vi "DiffDriveTrainSim_CreateKitbotSim_EstMass.vi"(5 "j_KgM2":dbl=1.0, 6 "MeasurementStdDev":T4, 8 "TrackWidth_M":dbl, 9 "Wheelsize":T1, 10 "ToughBoxMiniGear":T2, 11 "ToughBoxMiniMotor":T3) -> (0 "Size Coerced":bool, 3 "DiffDriveTrainSim":T5 {"m_Motor"."Jr_KgM2" format="%13.5p"; "m_Motor"."L_H" format="%13.5p"; "m_Motor"."Kt_NMPerAmp" format="%13.5p"; "m_Motor"."KvINV_RadPerSecPerVolt" format="%13.5p"; "m_Motor"."R_Ohms" format="%13.5p"; "m_Motor"."FreeSpeed_RadPerSec" format="%13.5p"; "m_Motor"."FreeCurrent_Amps" format="%13.5p"; "m_Motor"."StallCurrent_Amps" format="%13.5p"; "m_Motor"."StallTorque_NM" format="%13.5p"; "m_Motor"."nominalVoltage_Volts" format="%13.5p"})   [LabVIEW 2019, in "Trajectory_Library.lvlib"]
doc: "Create a sim for the standard FRC kitbot.\n\nThe mass of the robot is estimated at 25 pounds, converted to kg before use.\n \nInputs:\n - jKgMetersSquared -- The moment of inertia of the drivebase. This can be calculated using SysId.\n - motor -- The motors installed in the bot.\n - gearing -- The gearing reduction used.\n - wheelSize -- The wheel size.\n - trackWidth -- Width between left and right wheels - Meters\n - measurementStdDevs -- Standard deviations for measurements, in the form [x, y, heading, left velocity, right velocity, left distance, right distance]?. Can be null if no noise is desired. Gyro standard deviations of 0.0001 radians, velocity standard deviations of 0.05 m/s, and position measurement standard deviations of 0.005 meters are a reasonable starting point.\n\nOutputs:\n - OutDiffDriveTraimSim -- Updated data cluster.\n - SizeCoerced -- If TRUE, an error occured. Execution may continue"
uses:
  Trajectory_Library.lvlib
  TypeDef/DIFF_DRIVE_TRAIN_SIM.ctl
  TypeDef/LINEAR_SYSTEM.ctl
  <vilib>/Analysis/Matrix/Datatypes/RealMatrix.ctl
  TypeDef/DCMOTOR.CTL
  Enum/DIFF_DRIVE_ToughBoxMini_MotorChoice_ENUM.ctl
  Enum/DIFF_DRIVE_ToughBoxMini_GearChoice_ENUM.ctl
  Enum/DIFF_DRIVE_KitBot_WheelSize_ENUM.ctl
  <vilib>/Analysis/Matrix/NI_Matrix.lvlib
panel:
  # "<1, 1>"
  # "<States, 1>"
  # "<Outputs, 1>"
  # "<Inputs, 1>"
  # "<Outputs, 1>"
  # "<States,States>"
  # "<States,Inputs>"
  # "<Outputs,States>"
  # "<Outputs,Inputs>"
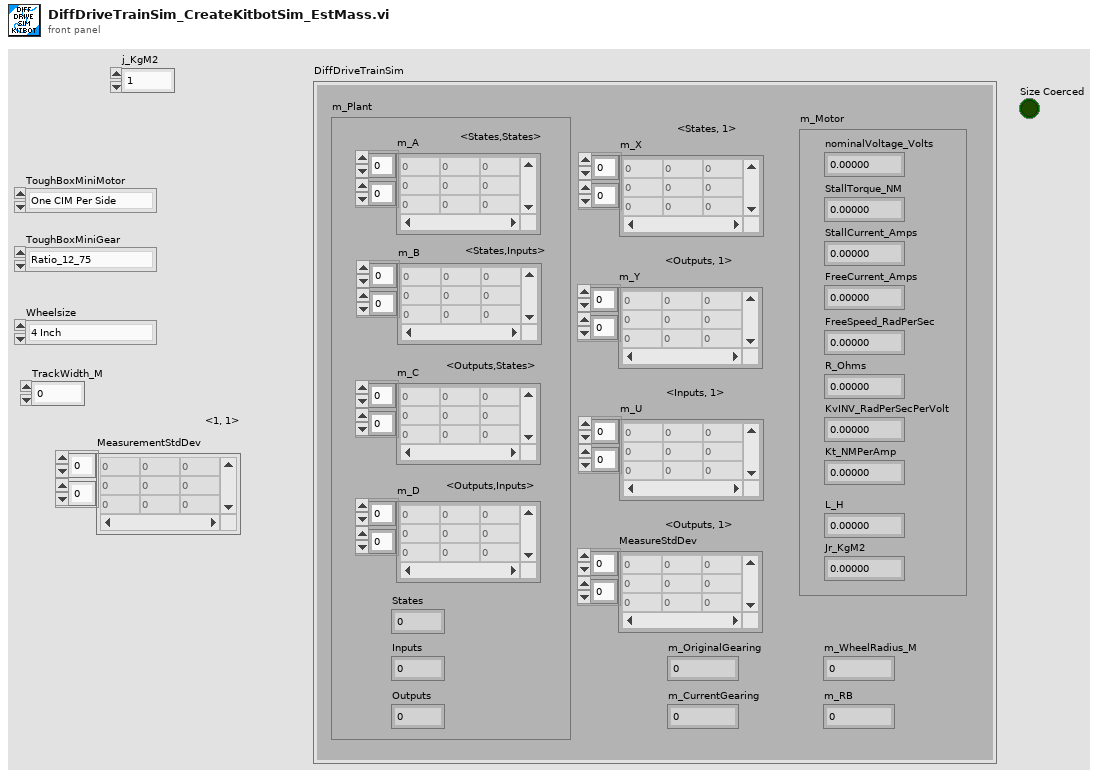
[diagram p1: front panel]
types:
  T1 = typedef "Trajectory_Library.lvlib/DIFF_DRIVE_KitBot_WheelSize_ENUM.ctl" = enum16{"4 Inch", "6 Inch", "8 Inch", "10 Inch"}
  T2 = typedef "Trajectory_Library.lvlib/DIFF_DRIVE_ToughBoxMini_GearChoice_ENUM.ctl" = enum16{"Ratio_12_75", "Ratio_10_71", "Ratio_8_45", "Ratio_7_31", "Ratio_5_95"}
  T3 = typedef "Trajectory_Library.lvlib/DIFF_DRIVE_ToughBoxMini_MotorChoice_ENUM.ctl" = enum16{"One CIM Per Side", "Two CIM Per Side", "One MiniCIM Per Side", "Two Mini CIM Per Side", "Two Falcon Per Side", "Two NEO Per Side"}
  T4 = typedef "NI_Matrix.lvlib/RealMatrix.ctl" = dbl[][]
  T5 = typedef "Trajectory_Library.lvlib/DIFF_DRIVE_TRAIN_SIM.ctl" = cluster{"m_Plant":T6, "m_X":T4, "m_Y":T4, "m_U":T4, "MeasureStdDev":T4, "m_Motor":T7, "m_OriginalGearing":dbl, "m_CurrentGearing":dbl, "m_WheelRadius_M":dbl, "m_RB":dbl}
  T6 = typedef "Trajectory_Library.lvlib/LINEAR_SYSTEM.ctl" = cluster{"m_A":T4, "m_B":T4, "m_C":T4, "m_D":T4, "States":i32, "Inputs":i32, "Outputs":i32}
  T7 = typedef "Trajectory_Library.lvlib/DCMOTOR.CTL" = cluster{"nominalVoltage_Volts":dbl, "StallTorque_NM":dbl, "StallCurrent_Amps":dbl, "FreeCurrent_Amps":dbl, "FreeSpeed_RadPerSec":dbl, "R_Ohms":dbl, "KvINV_RadPerSecPerVolt":dbl, "Kt_NMPerAmp":dbl, "L_H":dbl, "Jr_KgM2":dbl}
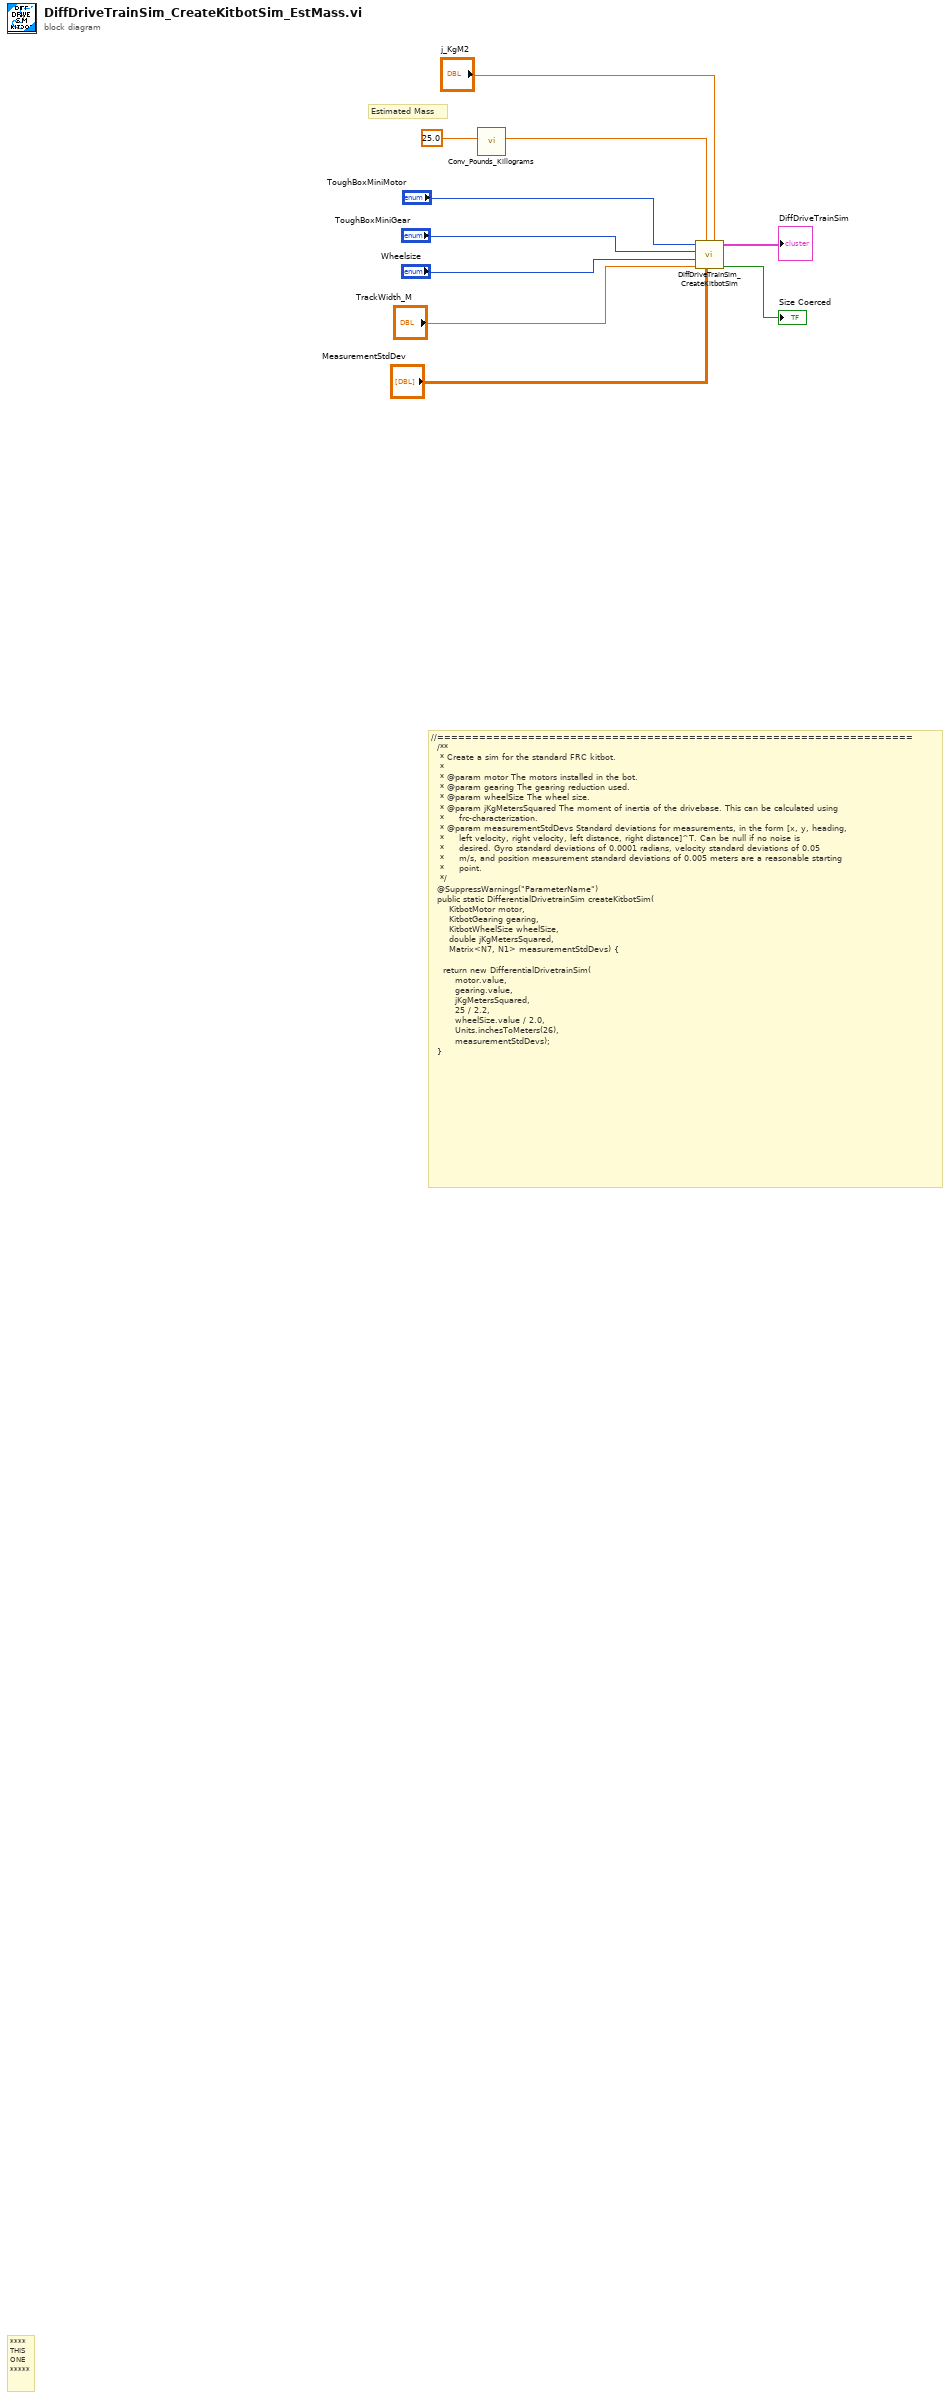
[diagram p0: block diagram]
diagram:
  # "Estimated Mass"
  # "//====================================================================\n  /**\n   * Create a sim for the standard FRC kitbot.\n   *\n   * @param motor The motors installed in the bot.\n   * @param gearing The gearing reduction used.\n   * @param wheelSize The wheel size.\n   * @param jKgMetersSquared The moment of inertia of the drivebase. This can be calculated using\n   *     frc-characterization.\n   * @param measurementStdDevs Standard deviations for measurements, in the form [x, y, heading,\n   *     left velocity, right velocity, left distance, right distance]^T. Can be null if no noise is\n   *     desired. Gyro standard deviations of 0.0001 radians, velocity standard deviations of 0.05\n   *     m/s, and position measurement standard deviations of 0.005 meters are a reasonable starting\n   *     point.\n   */\n  @SuppressWarnings(\"ParameterName\")\n  public static DifferentialDrivetrainSim createKitbotSim(\n      KitbotMotor motor,\n      KitbotGearing gearing,\n      KitbotWheelSize wheelSize,\n      double jKgMetersSquared,\n      Matrix<N7, N1> measurementStdDevs) {\n\n    return new DifferentialDrivetrainSim(\n        motor.value,\n        gearing.value,\n        jKgMetersSquared,\n        25 / 2.2,\n        wheelSize.value / 2.0,\n        Units.inchesToMeters(26),\n        measurementStdDevs);\n  }"
  # "****\nTHIS\nONE\n*****"
  n1 = call "Conv_Pounds_Killograms.vi"("Pounds"=25.0 ("x")) -> ("Killograms"=w3:dbl)  [unwired: 10 in]
  n2 = call "DiffDriveTrainSim_CreateKitbotSim.vi"("j_KgM2"="j_KgM2", "MeasurementStdDev"="MeasurementStdDev", "Mass_Kg"=w3, "TrackWidth_M"="TrackWidth_M", "Wheelsize"="Wheelsize", "ToughBoxMiniGear"="ToughBoxMiniGear", "ToughBoxMiniMotor"="ToughBoxMiniMotor") -> ("Size Coerced"=→"Size Coerced":bool, "DiffDriveTrainSim"=→"DiffDriveTrainSim":T5)  [unwired: 3 in]
